vi "Stream with autorestart and data checking.vi"() -> ()   [LabVIEW 2020]
panel:
  in  "Disable Autorecovery":bool
  out "Flagged Row":i32
  in  "STREAM_BUFFER_SIZE_BYTES":i32=4096
  out "Library":dbl format="%.4g"
  out "Firmware":dbl format="%.4g"
  out "Hardware":dbl format="%.4g"
  out "Start/Stop log":string[](array[string])
  in  "#Seconds on Graph":dbl=1.0 format="%.2f"
  out "Actual SampleRate (Hz)":dbl format="%.3f"
  out "NumAddresses":i32
  in  "STREAM_RESOLUTION_INDEX":i32
  in  "STREAM_SETTLING_US":i32
  in  "AIN_ALL_RANGE":dbl=10.0 format="%.3f"
  out "ScansPerRead":i32
  out "ConnectionType Out":i32
  out "DeviceType Out":i32
  in  "Identifier":string="192.168.1.247"
  in  "ConnectionType":string="wifi"
  in  "DeviceType":string="t7"
  out "DeviceScanBacklog":i32
  out "LJMScanBacklog":i32
  out "Data":dbl[][](array[numeric]) format="%.3f"
  out "Waveform Graph":dbl[](graph)
  in  "Scan List":i32[](array[numeric])=[0, 0, 4897, 4898]
  out "# of iterations":i32
  in  "Scan Rate (Hz)":dbl=100.0 format="%.3f"
  in  "stop":bool
  out "Error Message":string
  # "Jumper VS to AIN0!"
  # "To remove an element, right-click\non it, select Data Operations =>\nRemove Element.\n\nTo empty an array, right-click\nnear the edge, select Data\nOperations => Empty Array.\n\nOther useful operations:  From the\nOperate menu are \"Make Current\nValues Default\" and \"Reinitialize\nTo Default\"."
  # "32768 max"
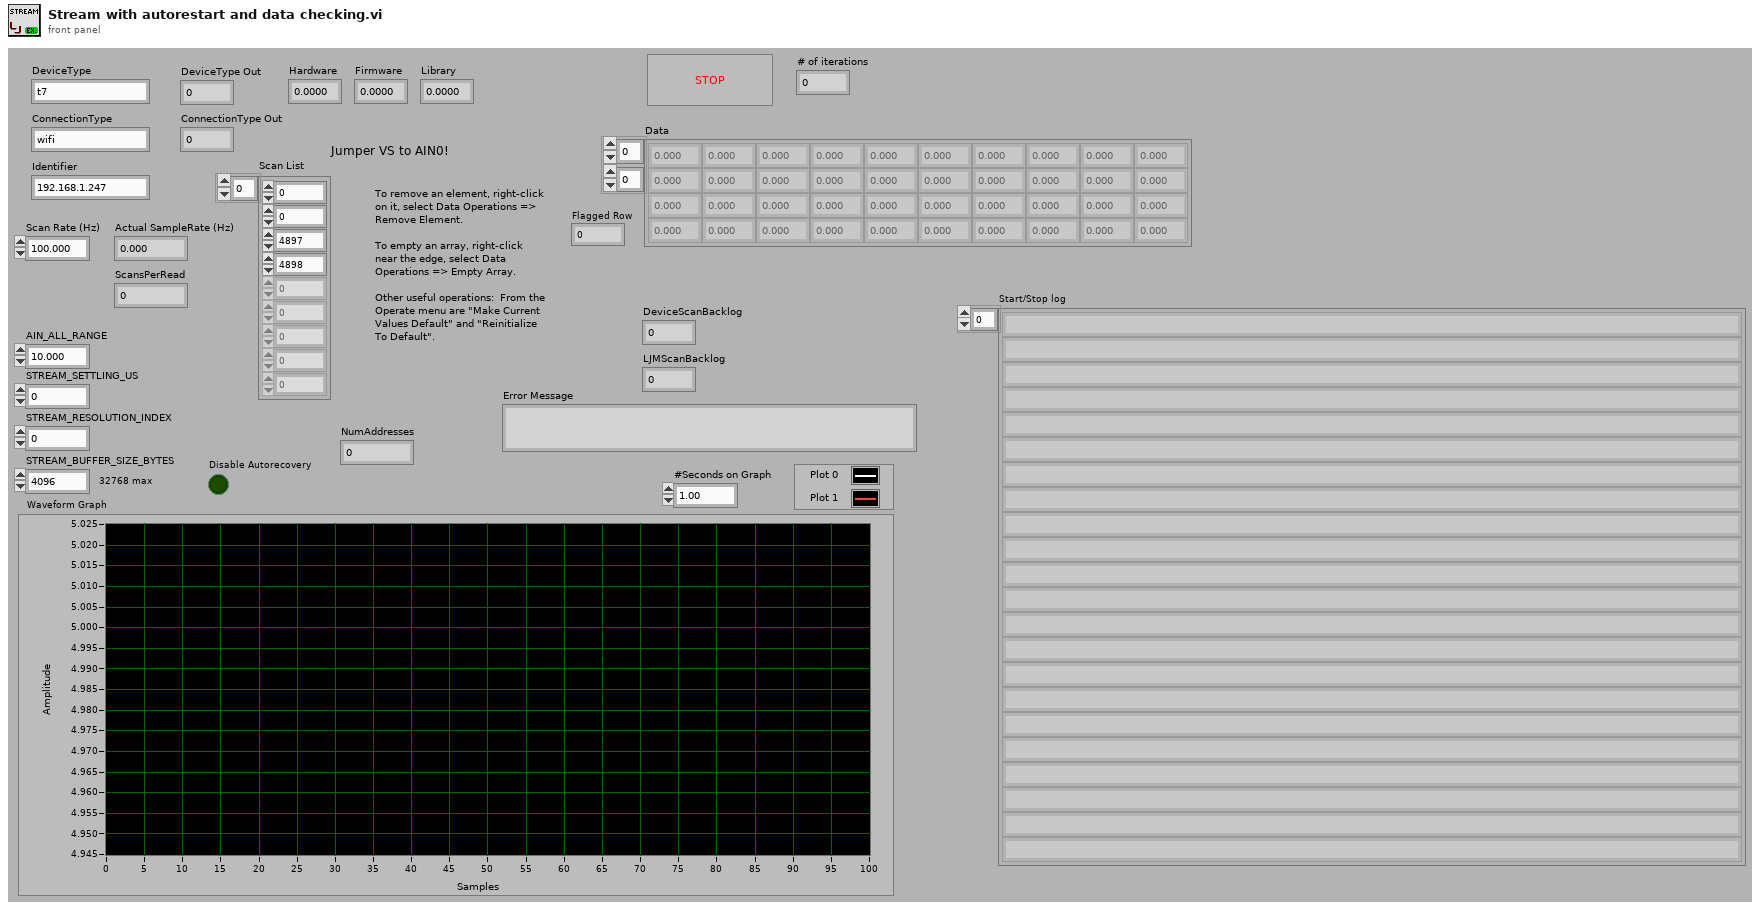
[diagram p1: front panel]
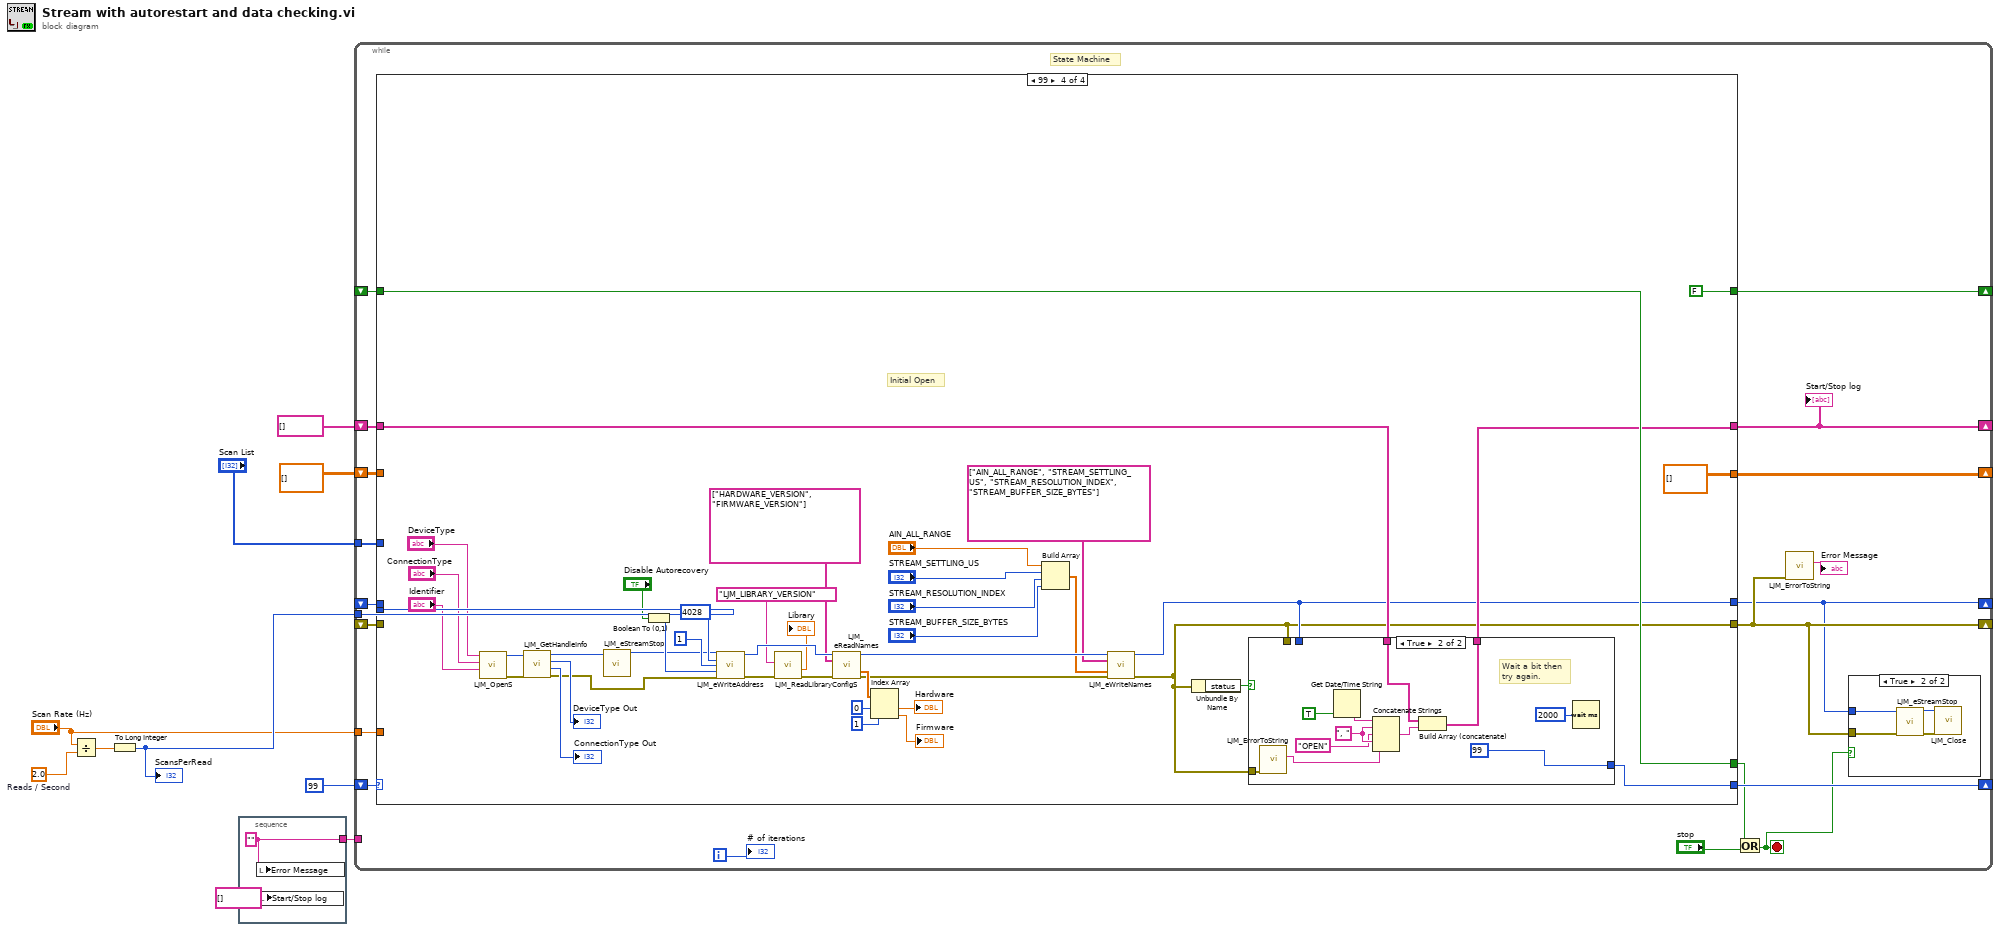
[diagram p0: block diagram]
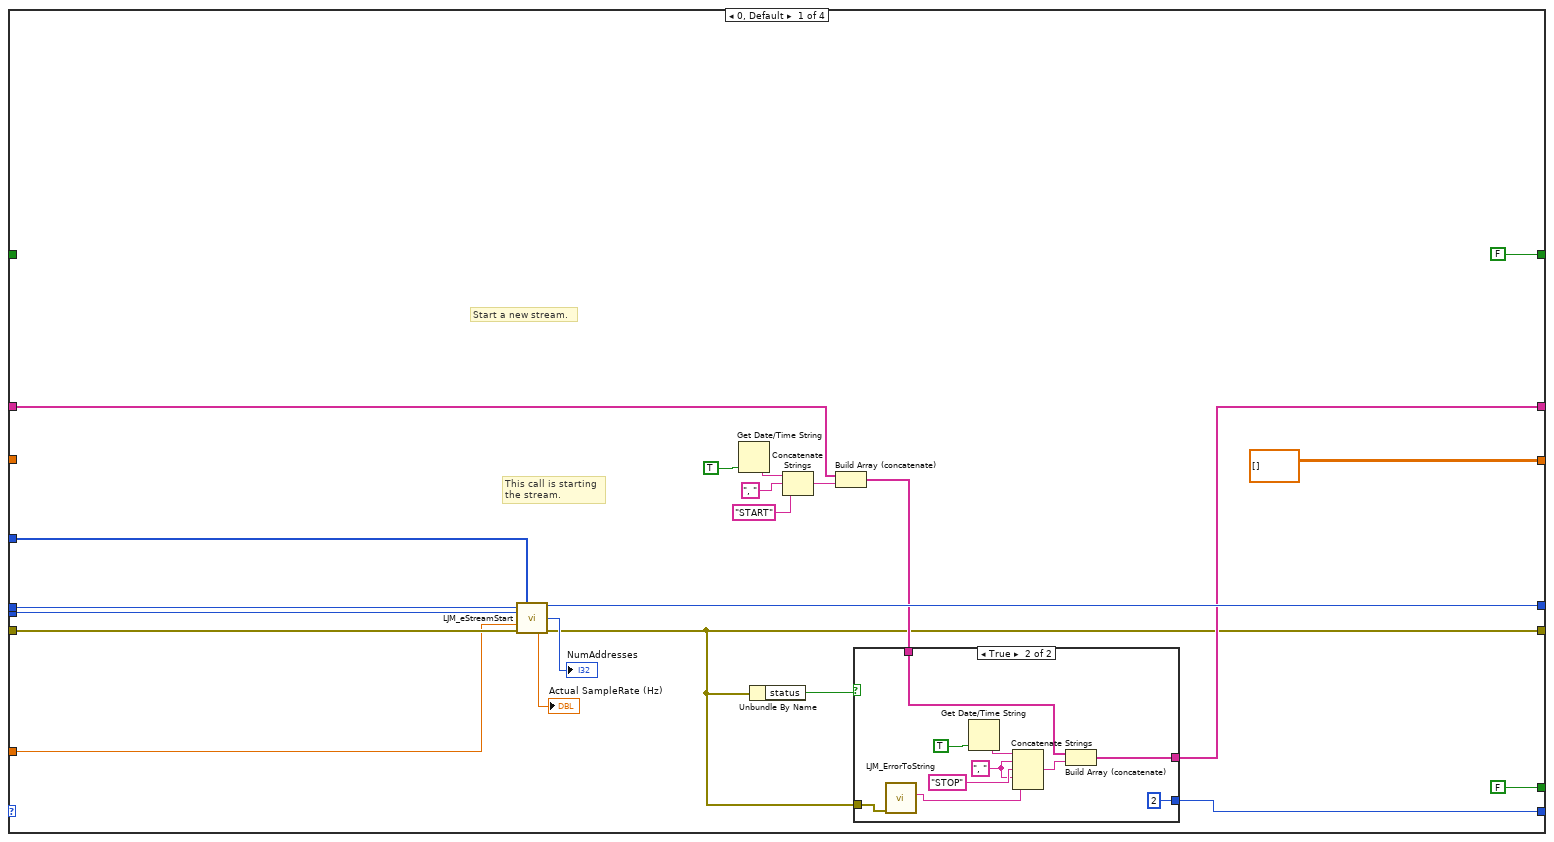
[diagram p3: hidden frame]
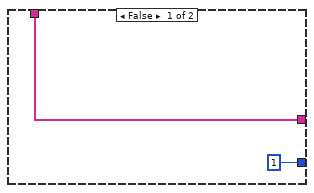
[diagram p4: hidden frame]
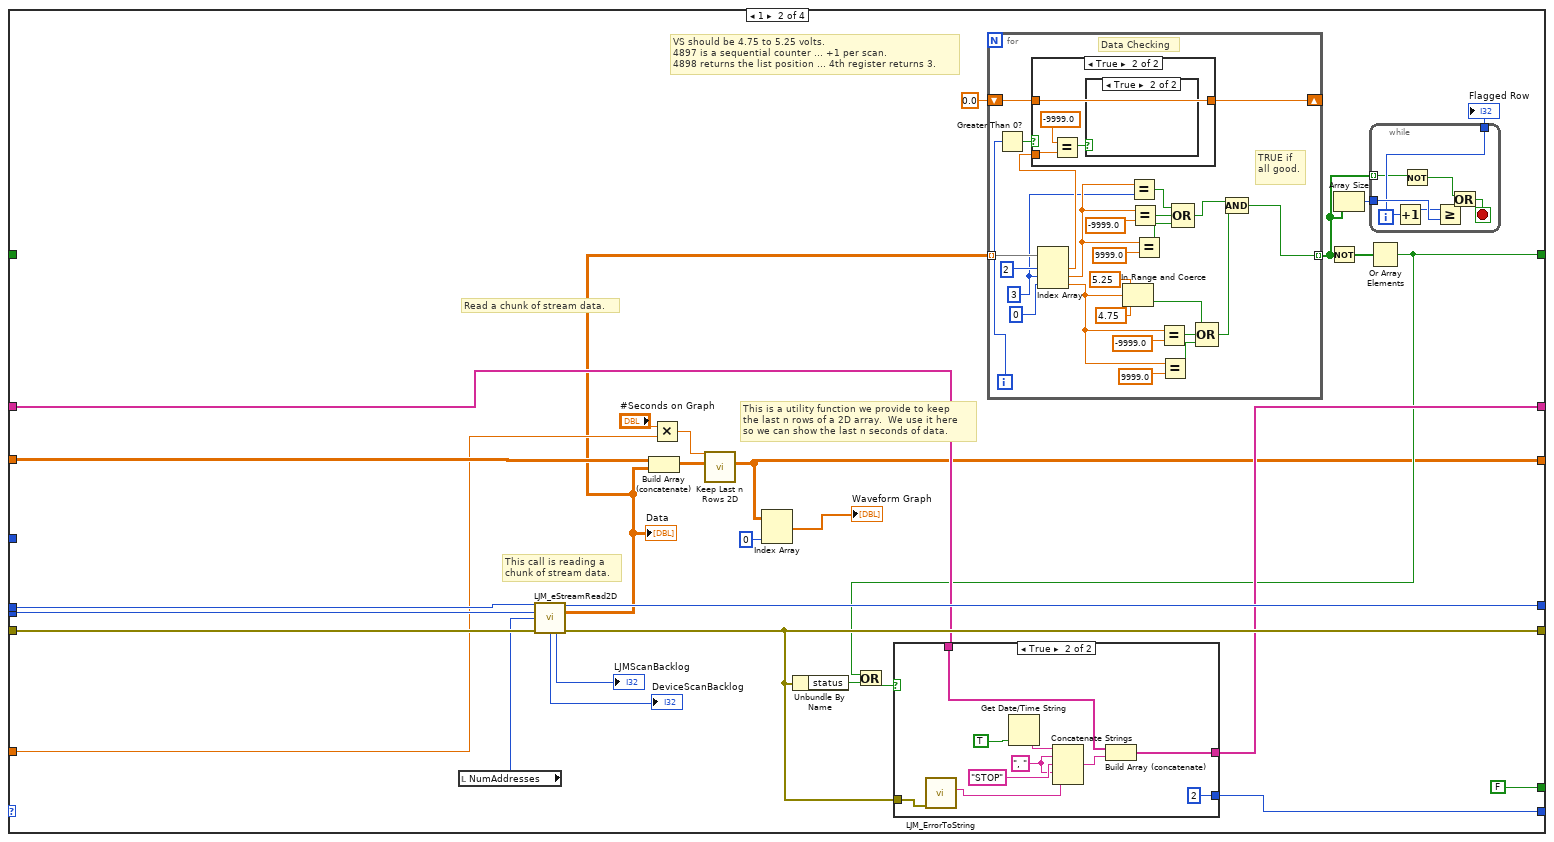
[diagram p5: hidden frame]
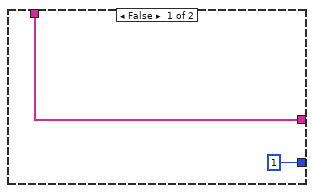
[diagram p8: hidden frame]
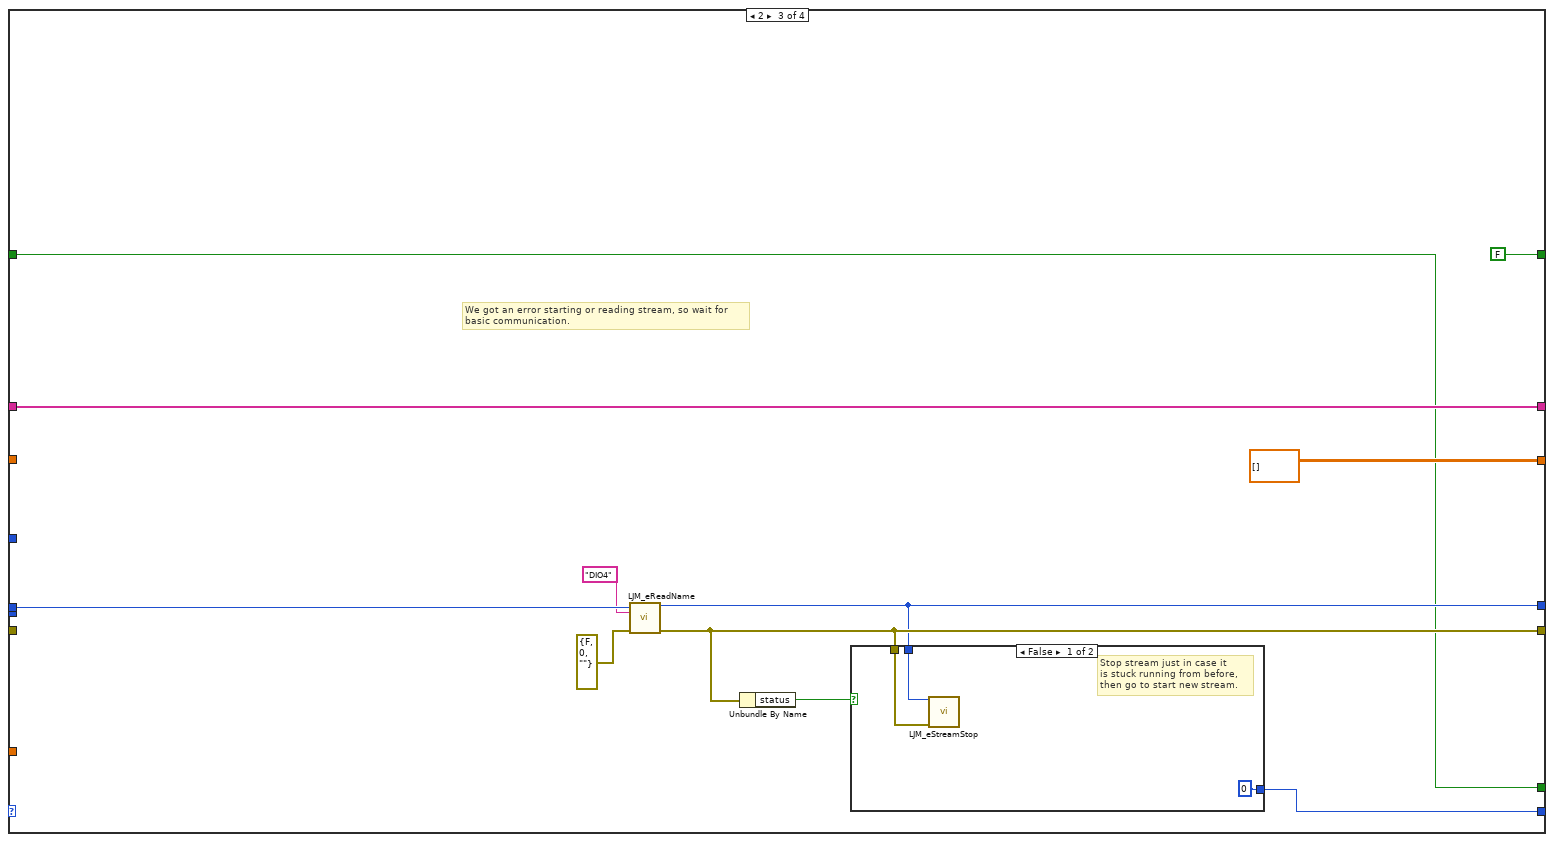
[diagram p9: hidden frame]
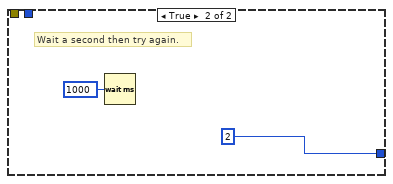
[diagram p10: hidden frame]
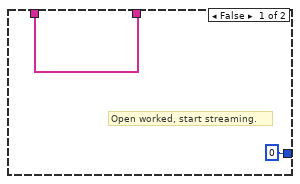
[diagram p11: hidden frame]
diagram:
  w9 = 2.0  # Reads / Second
  n1 = Divide(x="Scan Rate (Hz)", y=w9) -> (x/y=w8:dbl)
  n2 = To Long Integer(number=w8) -> (32bit integer=w7:i32)
  "ScansPerRead" <- w7
  n3 = stacked-sequence {
    tunnel: [w11] -> w1
    frame #0 {
      w11 = "" ("Error Message")
      n4 = local write "Error Message"(w11) -> ()
      n5 = local write "Start/Stop log"(string[] [] ("Start/Stop log")) -> ()
    }
  }
  n6 = while {
    tunnel: w7 -> [w30]
    tunnel: "Scan List" -> [w28]
    tunnel: "Scan Rate (Hz)" -> [w27]
    shift-right: [w22] -> _
    shift-left: 99 -> [w26]
    shift-right: [w13] -> _
    shift-left: _ -> [w31]
    shift-right: [w25] -> _
    shift-left: dbl[][] [] ("Last n Rows") -> [w24]
    shift-right: [w19] -> _
    shift-left: string[] [] -> [w21]
    shift-right: [w12] -> _
    shift-left: _ -> [w29]
    shift-right: [w18] -> _
    shift-left: _ -> [w15]
    tunnel: w1 -> [_]
    i -> [w23]
    stop <- w14 stop-if-true
    # "State Machine"
    n7 = case shown="99" w26 {
      tunnel: w31 -> [w57 w92 _ _]
      tunnel: w30 -> [w56 w90 _ _]
      tunnel: w29 -> [w55 w91 w159 _]
      tunnel: w28 -> [w54 _ _ _]
      tunnel: w27 -> [w51 w89 _ _]
      tunnel: [w38 w86 w154 w168] -> w13
      tunnel: [dbl[][] [] ("Last n Rows") w72 dbl[][] [] ("Last n Rows") dbl[][] [] ("Last n Rows")] -> w25
      tunnel: w24 -> [_ w93 _ _]
      tunnel: [w39 w83 w155 w205] -> w22
      tunnel: [w49 w87 w152 w169] -> w12
      tunnel: [w41 w84 w151 w200] -> w19
      tunnel: w21 -> [w40 w85 w151 w201]
      tunnel: [FALSE w77 FALSE FALSE] -> w18
      tunnel: [FALSE FALSE w149 w202] -> w16
      tunnel: w15 -> [_ _ w149 w202]
      frame 0, Default {
        # "Start a new stream."
        # "This call is starting\nthe stream."
        n8 = call "LJM_eStreamStart.vi"("Handle In"=w55, "aScanList"=w54, "ScansPerRead"=w56, "ScanRate"=w51, "error in"=w57) -> ("Handle Out"=w49:i32, "NumReadAddresses"=→"NumAddresses":i32, "Actual SampleRate"=→"Actual SampleRate (Hz)":dbl, "error out"=w38:errorcluster)  [unwired: 5 in, 2 out]
        n9 = Get Date/Time String(want seconds? (F)=TRUE) -> (time string=w44:string)  [unwired: 2 in, 1 out]
        n10 = Unbundle By Name(w38) -> ("status"=w43:bool)
        n11 = Concatenate Strings(w44, ", " ("string"), "START" ("string")) -> (w47:string)
        n12 = Build Array (concatenate)(w40, w47) -> (w42:string[])
        n13 = case shown="True" w43 {
          tunnel: w42 -> [w59 w65]
          tunnel: [w59 w64] -> w41
          tunnel: w38 -> [_ w62]
          tunnel: [1 2] -> w39
          frame False {
          }
          frame True {
            w63 = ", " ("string")
            n14 = call "LJM_ErrorToString.vi"("error in"=w62) -> ("String"=w61:string)  [unwired: 10 in]
            n15 = Get Date/Time String(want seconds? (F)=TRUE) -> (time string=w66:string)  [unwired: 2 in, 1 out]
            n16 = Concatenate Strings(w66, w63, "STOP" ("string"), w63, w61) -> (w68:string)
            n17 = Build Array (concatenate)(w65, w68) -> (w64:string[])
          }
        }
      }
      frame 1 {
        # "VS should be 4.75 to 5.25 volts.\n4897 is a sequential counter ... +1 per scan.\n4898 returns the list position ... 4th register returns 3."
        # "This call is reading a\nchunk of stream data."
        # "This is a utility function we provide to keep\nthe last n rows of a 2D array.  We use it here\nso we can show the last n seconds of data."
        # "Read a chunk of stream data."
        n18 = local read "NumAddresses"() -> (w88:i32)
        n19 = call "LJM_eStreamRead2D.vi"("Handle In"=w91, "ScansPerRead"=w90, "NumAddresses"=w88, "error in"=w92) -> ("Handle Out"=w87:i32, "aData Out"=w82:dbl[][], "DeviceScanBacklog"=→"DeviceScanBacklog":i32, "LJMScanBacklog"=→"LJMScanBacklog":i32, "error out"=w86:errorcluster)  [unwired: 7 in]
        "Data" <- w82
        n20 = Build Array (concatenate)(w93, w82) -> (w97:dbl[][])
        n21 = Multiply(x="#Seconds on Graph", y=w89) -> (x*y=w98:dbl)
        n22 = call "Keep Last n Rows 2D.vi"("Array"=w97, "# Rows to Keep"=w98) -> ("Last n Rows"=w72:dbl[][])  [unwired: 9 in]
        n23 = Index Array(array=w72, index (col)=0 ("disabled index (col)")) -> (element=→"Waveform Graph":dbl[])  [unwired: 1 in]
        n24 = Unbundle By Name(w86) -> ("status"=w78:bool)
        n25 = for {
          tunnel: w82 -> [w131] mode=indexing
          shift-right: [w124] -> _
          shift-left: 0.0 -> [w122]
          tunnel: [w121] -> w75 mode=indexing
          i -> [w125]
          w106 = 3 ("index")
          # "Data Checking"
          # "TRUE if\nall good."
          n26 = Greater Than 0?(x=w125) -> (x > 0?=w126:bool)
          n27 = Index Array(array=w131, index #1=2 ("index (row)"), index #2=w106, index #3=0 ("index")) -> (element #1=w123:dbl, element #2=w109:dbl, element #3=w108:dbl)
          n28 = case shown="True" w126 {
            tunnel: [w132 w133] -> w124
            tunnel: w123 -> [w132 w135]
            tunnel: w122 -> [_ w133]
            frame False {
            }
            frame True {
              n29 = Equal?(x=-9999.0, y=w135) -> (x = y?=w134:bool)
              n30 = case shown="True" w134 {
                frame False {
                }
                frame True {
                }
              }
            }
          }
          n31 = In Range and Coerce(upper limit=5.25 ("lower limit"), x=w108, lower limit=4.75 ("upper limit")) -> (In Range?=w117:bool)  [unwired: 1 out]
          n32 = Equal?(x=w109, y=w106) -> (x = y?=w112:bool)
          n33 = Equal?(x=w109, y=-9999.0) -> (x = y?=w113:bool)
          n34 = Equal?(x=w109, y=9999.0) -> (x = y?=w110:bool)
          n35 = Equal?(x=w108, y=-9999.0) -> (x = y?=w116:bool)
          n36 = Equal?(x=w108, y=9999.0) -> (x = y?=w115:bool)
          n37 = Compound Arithmetic op=OR(w112, w113, w110) -> (w107:bool)
          n38 = Compound Arithmetic op=OR(w117, w116, w115) -> (w114:bool)
          n39 = Compound Arithmetic op=AND(w107, w114) -> (w121:bool)
        }
        n40 = Not(x=w75) -> (.not. x?=w80:bool[])
        n41 = Array Size(array=w75) -> (size(s)=w74:i32)
        n42 = while {
          tunnel: w75 -> [w100] mode=indexing
          tunnel: w74 -> [w103]
          tunnel: [w102] -> w73
          i -> [w102]
          stop <- w104 stop-if-true
          n43 = Increment(x=w102) -> (x+1=w101:i32)
          n44 = Not(x=w100) -> (.not. x?=w99:bool)
          n45 = Greater Or Equal?(x=w101, y=w103) -> (x >= y?=w105:bool)
          n46 = Or(x=w99, y=w105) -> (x .or. y?=w104:bool)
        }
        "Flagged Row" <- w73
        n47 = Or Array Elements(Boolean array=w80) -> (logical OR=w77:bool)
        n48 = Or(x=w77, y=w78) -> (x .or. y?=w79:bool)
        n49 = case shown="True" w79 {
          tunnel: w85 -> [w138 w144]
          tunnel: [w138 w143] -> w84
          tunnel: w86 -> [_ w141]
          tunnel: [1 2] -> w83
          frame False {
          }
          frame True {
            w142 = ", " ("string")
            n50 = call "LJM_ErrorToString.vi"("error in"=w141) -> ("String"=w140:string)  [unwired: 10 in]
            n51 = Get Date/Time String(want seconds? (F)=TRUE) -> (time string=w145:string)  [unwired: 2 in, 1 out]
            n52 = Concatenate Strings(w145, w142, "STOP" ("string"), w142, w140) -> (w147:string)
            n53 = Build Array (concatenate)(w144, w147) -> (w143:string[])
          }
        }
      }
      frame 2 {
        # "We got an error starting or reading stream, so wait for\nbasic communication."
        n54 = call "LJM_eReadName.vi"("Handle In"=w159, "Name"="DIO4", "error in"=errorcluster {"status"=FALSE, "code"=0, "source"=""}) -> ("Handle Out"=w152:i32, "error out"=w154:errorcluster)  [unwired: 10 in, 1 out]
        n55 = Unbundle By Name(w154) -> ("status"=w156:bool)
        n56 = case shown="False" w156 {
          tunnel: [0 2] -> w155
          tunnel: w152 -> [w161 _]
          tunnel: w154 -> [w160 _]
          frame False {
            # "Stop stream just in case it\nis stuck running from before,\nthen go to start new stream."
            n57 = call "LJM_eStreamStop.vi"("Handle In"=w161, "error in"=w160) -> ()  [unwired: 12 in, 2 out]
          }
          frame True {
            # "Wait a second then try again."
            n58 = Wait (ms)(milliseconds to wait=u32 1000) -> ()  [unwired: 1 out]
          }
        }
      }
      frame 99 {
        # "Initial Open"
        n59 = call "LJM_OpenS.vi"("Identifier"="Identifier", "ConnectionType"="ConnectionType", "DeviceType"="DeviceType") -> ("error out"=w170:errorcluster, "Handle"=w173:i32)  [unwired: 7 in]
        n60 = call "LJM_GetHandleInfo.vi"("error in"=w170, "Handle In"=w173) -> ("error out"=w165:errorcluster, "ConnectionType"=→"ConnectionType Out":i32, "DeviceType"=→"DeviceType Out":i32, "Handle Out"=w167:i32)  [unwired: 2 in, 4 out]
        n61 = call "LJM_eStreamStop.vi"("Handle In"=w167) -> ("Handle Out"=w166:i32)  [unwired: 13 in, 1 out]
        n62 = Boolean To (0,1)(Boolean="Disable Autorecovery") -> (0, 1=w199:i16)
        n63 = call "LJM_eWriteAddress.vi"("Handle In"=w166, "Address"=4028, "Type"=1, "Value"=w199, "error in"=w165) -> ("Handle Out"=w194:i32, "error out"=w195:errorcluster)  [unwired: 9 in]
        n64 = call "LJM_ReadLibraryConfigS.vi"("error in"=w195, "Parameter"="LJM_LIBRARY_VERSION") -> ("error out"=w185:errorcluster, "Value"=→"Library":dbl)  [unwired: 8 in]
        n65 = call "LJM_eReadNames.vi"("Handle In"=w194, "aNames"=string[] ["HARDWARE_VERSION", "FIRMWARE_VERSION"], "error in"=w185) -> ("Handle Out"=w187:i32, "aValuesOut"=w189:dbl[], "error out"=w186:errorcluster)  [unwired: 9 in, 1 out]
        n66 = Index Array(array=w189, index #1=0 ("index"), index #2=1 ("index")) -> (element #1=→"Hardware":dbl, element #2=→"Firmware":dbl)
        n67 = Build Array("AIN_ALL_RANGE", "STREAM_SETTLING_US", "STREAM_RESOLUTION_INDEX", "STREAM_BUFFER_SIZE_BYTES") -> (w179:dbl[])
        n68 = call "LJM_eWriteNames.vi"("Handle In"=w187, "aNames"=string[] ["AIN_ALL_RANGE", "STREAM_SETTLING_US", "STREAM_RESOLUTION_INDEX", "STREAM_BUFFER_SIZE_BYTES"], "aValuesIn"=w179, "error in"=w186) -> ("Handle Out"=w169:i32, "error out"=w168:errorcluster)  [unwired: 9 in, 1 out]
        n69 = Unbundle By Name(w168) -> ("status"=w206:bool)
        n70 = case shown="True" w206 {
          tunnel: [0 99] -> w205
          tunnel: w169 -> [_ _]
          tunnel: w168 -> [_ _]
          tunnel: w201 -> [w207 w211]
          tunnel: [w207 w210] -> w200
          tunnel: w168 -> [_ w209]
          frame False {
            # "Open worked, start streaming."
          }
          frame True {
            w216 = ", " ("string")
            # "Wait a bit then\ntry again."
            n71 = call "LJM_ErrorToString.vi"("error in"=w209) -> ("String"=w217:string)  [unwired: 10 in]
            n72 = Get Date/Time String(want seconds? (F)=TRUE) -> (time string=w215:string)  [unwired: 2 in, 1 out]
            n73 = Concatenate Strings(w215, w216, "OPEN" ("string"), w216, w217) -> (w213:string)
            n74 = Build Array (concatenate)(w211, w213) -> (w210:string[])
            n75 = Wait (ms)(milliseconds to wait=u32 2000) -> ()  [unwired: 1 out]
          }
        }
      }
    }
    "Start/Stop log" <- w19
    n76 = Or(x=w16, y="stop") -> (x .or. y?=w14:bool)
    n77 = call "LJM_ErrorToString.vi"("error in"=w13) -> ("String"=→"Error Message":string)  [unwired: 10 in]
    n78 = case shown="True" w14 {
      tunnel: w13 -> [_ w32]
      tunnel: w12 -> [_ w33]
      frame False {
      }
      frame True {
        n79 = call "LJM_eStreamStop.vi"("Handle In"=w33, "error in"=w32) -> ("Handle Out"=w34:i32, "error out"=w35:errorcluster)  [unwired: 12 in]
        n80 = call "LJM_Close.vi"("error in"=w35, "Handle"=w34) -> ()  [unwired: 9 in, 1 out]
      }
    }
    "# of iterations" <- w23
  }
